vi "UDP_Packet-Bin.vi"(9 "IN_BIN":string, 11 "IN_Packet":T1 {"Command" format="%.0x"}) -> (1 "OUT_Packet":T1 {"Command" format="%.0x"}, 3 "OUT_BIN":string)   [LabVIEW 2017]
uses:
  UDP_Packet.ctl
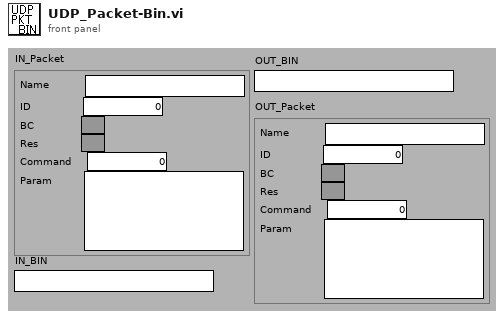
[diagram p1: front panel]
types:
  T1 = typedef "UDP_Packet.ctl" = cluster{"Name":string, "ID":u32, "BC":bool, "Res":bool, "Command":u32, "Param":string}
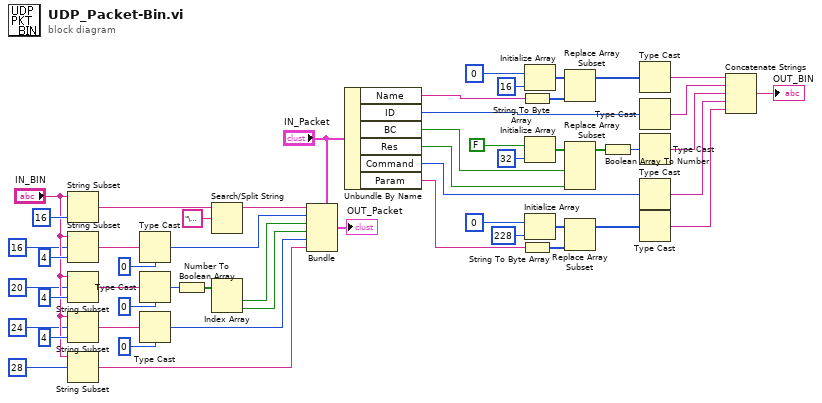
[diagram p0: block diagram]
diagram:
  n1 = String Subset(string="IN_BIN", length (rest)=16 ("length (rest)")) -> (substring=w10:string)  [unwired: 1 out]
  n2 = String Subset(string="IN_BIN", offset (0)=16, length (rest)=4 ("length (rest)")) -> (substring=w9:string)
  n3 = String Subset(string="IN_BIN", offset (0)=20, length (rest)=4 ("length (rest)")) -> (substring=w8:string)
  n4 = String Subset(string="IN_BIN", offset (0)=24, length (rest)=4 ("length (rest)")) -> (substring=w7:string)
  n5 = String Subset(string="IN_BIN", offset (0)=28) -> (substring=w6:string)  [unwired: 1 out]
  n6 = Type Cast(type=u32 0 ("dimension size"), x=w9) -> (*(type *) &x=w25:u32)
  n7 = Type Cast(type=u32 0 ("dimension size"), x=w8) -> (*(type *) &x=w20:u32)
  n8 = Type Cast(type=u32 0 ("dimension size"), x=w7) -> (*(type *) &x=w22:u32)
  n9 = Number To Boolean Array(number=w20) -> (Boolean array=w19:bool[])
  n10 = Search/Split String(string=w10, search string/char (-)="\u0000") -> (substring before match=w26:string)  [unwired: 3 out]
  n11 = Index Array(array=w19) -> (element #1=w18:bool, element #2=w17:bool)  [unwired: 2 in]
  n12 = Bundle(cluster="IN_Packet", "Name"=w26, "ID"=w25, "BC"=w18, "Res"=w17, "Command"=w22, "Param"=w6) -> (→"OUT_Packet":T1)
  n13 = Unbundle By Name("IN_Packet") -> ("Name"=w53:string, "ID"=w41:u32, "BC"=w46:bool, "Res"=w45:bool, "Command"=w40:u32, "Param"=w35:string)
  n14 = String To Byte Array(string=w53) -> (unsigned byte array=w50:u8[])
  n15 = String To Byte Array(string=w35) -> (unsigned byte array=w39:u8[])
  n16 = Initialize Array(u8 0 ("dimension size"), 16 ("dimension size")) -> (w51:u8[])
  n17 = Initialize Array(FALSE, 32 ("dimension size")) -> (w49:bool[])
  n18 = Initialize Array(u8 0 ("dimension size"), 228 ("dimension size")) -> (w38:u8[])
  n19 = Replace Array Subset(array=w51, new element=w50) -> (w42:u8[])  [unwired: 1 in]
  n20 = Replace Array Subset(array=w49, new element #1=w46, new element #2=w45) -> (w44:bool[])  [unwired: 2 in]
  n21 = Replace Array Subset(array=w38, new element=w39) -> (w34:u8[])  [unwired: 1 in]
  n22 = Boolean Array To Number(Boolean array=w44) -> (number=w43:u32)
  n23 = Type Cast(x=w42) -> (*(type *) &x=w33:string)  [unwired: 1 out]
  n24 = Type Cast(x=w41) -> (*(type *) &x=w32:string)  [unwired: 1 out]
  n25 = Type Cast(x=w43) -> (*(type *) &x=w31:string)  [unwired: 1 out]
  n26 = Type Cast(x=w40) -> (*(type *) &x=w30:string)  [unwired: 1 out]
  n27 = Type Cast(x=w34) -> (*(type *) &x=w29:string)  [unwired: 1 out]
  n28 = Concatenate Strings(w33, w32, w31, w30, w29) -> (→"OUT_BIN":string)
